vi "Global - Monitoring Variables.vi"() -> ()   [LabVIEW 2015]
panel:
  in  "Safe Mode":refnum<k4> caption="安全模式"
  in  "Live Channels":string[](array[string]) caption="直播通道"
  out "Initial Scan":i64 caption="初始扫描周期"
  out "Initial Timestamp":timestamp caption="初始时间标识"
  out "Drive Space":dbl caption="驱动器空间"
  out "Buffer Backlog":dbl caption="缓冲区积压"
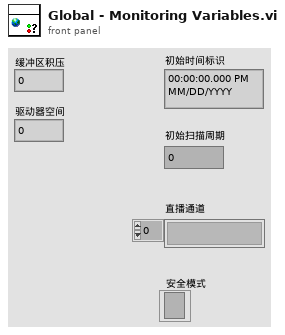
[diagram p1: front panel]
diagram:
